vi "Optic Spectrometer.vi"() -> ()   [LabVIEW 2019]
uses:
  <vilib>/DAQmx/write.llb/DAQmx Write (Digital 1D Bool 1Chan 1Samp).vi
  <vilib>/Analysis/baseanly.llb/Mean (DBL).vi
  <vilib>/DAQmx/create/channels.llb/DAQmx Create Channel (DO-Digital Output).vi
  <vilib>/DAQmx/miscellaneous.llb/DAQmx Fill In Error Info.vi
  <vilib>/Analysis/NI_AALBase.lvlib
panel:
  out "End Process":bool
  in  "States":bool[](array[boolean])
  in  "Tab Control":T1(tab)
  out "Gain":dbl=15.0 format="%#_13g"
  in  "Reverse":bool
  in  "Signal Polarity":u16(ring)=1 items=["Module Value", "Real Value"]
  in  "Background Color":u32(colorbox)=16448250
  in  "Plot Color":u32(colorbox)
  in  "Digital Port for Stepper motor":tag="Dev2/port0/line0:3"
  in  "Lamp Spectrum Measuring":bool
  in  "Device name":tag="Dev2"
  in  "Lamp DATA":path=path "C:/Users/Zaza/Google Drive/Projects/Optic Spectrometer/Results/Spectrs Data/Calibrate/250W lamp/IK-5-H1-0.2.txt" caption="Filename"
  in  "Save":bool=TRUE
  in  "Grid":enum32{"Radio Selection 1", "Radio Selection 2"}(radio)=enum."Radio Selection 2"
  in  "File Name":string="Name"
  out "Wavelength[um]":dbl
  out "Baraban":dbl
  in  "Start":dbl=120.0 format="%#_13g"
  in  "Stop":dbl=800.0 format="%#_13g"
  in  "Speed":dbl=100.0
  out "Original Curve":cluster{dbl, dbl}[](graph)=[{0.98, 0.594256}, {0.982, 0.591387}, {0.984, 0.592344}, {0.986, 0.596807}, {0.988, 0.59872}, {0.99, 0.60669}, {0.992, 0.611472}, {0.994, 0.619761}, {0.996, 0.628688}, {0.998, 0.640165}, {1.0, 0.650366}, {1.002, 0.659612}, {1.004, 0.675233}, {1.006, 0.684479}, {1.008, 0.698506}, {1.01, 0.706795}, {1.012, 0.719866}, {1.014, 0.733575}, {1.016, 0.747284}, {1.018, 0.762587}, {1.02, 0.771513}, {1.022, 0.782034}, {1.024, 0.787772}, {1.026, 0.8018}, {1.028, 0.812002}, {1.03, 0.825073}, {1.032, 0.838463}, {1.034, 0.84707}, {1.036, 0.854403}, {1.038, 0.863011}, {1.04, 0.88182}, {1.042, 0.898398}, {1.044, 0.907325}, {1.046, 0.915614}, {1.048, 0.923584}, {1.05, 0.934424}, {1.052, 0.951639}, {1.054, 0.966942}, {1.056, 0.971724}, {1.058, 0.980651}, {1.06, 0.993084}, {1.062, 1.006793}, {1.064, 1.01827}, {1.066, 1.024008}, {1.068, 1.034848}, {1.07, 1.041862}, {1.072, 1.053339}, {1.074, 1.060034}, {1.076, 1.073105}, {1.078, 1.079162}, {1.08, 1.085857}, {1.082, 1.096378}, {1.084, 1.102116}, {1.086, 1.11168}, {1.088, 1.121563}, {1.09, 1.131765}, {1.092, 1.139098}, {1.094, 1.141011}, {1.096, 1.140054}, {1.098, 1.144518}, {1.1, 1.139735}, {1.102, 1.136866}, {1.104, 1.128896}, {1.106, 1.117738}, {1.108, 1.106579}, {1.11, 1.105304}, {1.112, 1.106898}, {1.114, 1.102435}, {1.116, 1.099247}, {1.118, 1.096059}, {1.12, 1.099566}, {1.122, 1.104985}, {1.124, 1.110086}, {1.126, 1.116462}, {1.128, 1.113593}, {1.13, 1.119651}, {1.132, 1.126983}, {1.134, 1.131765}, {1.136, 1.141011}, {1.138, 1.143242}, {1.14, 1.148024}, {1.142, 1.154401}, {1.144, 1.16779}, {1.146, 1.181499}, {1.148, 1.19457}, {1.15, 1.206047}, {1.152, 1.20254}, {1.154, 1.209554}, {1.156, 1.207004}, {1.158, 1.207004}, {1.16, 1.207004}, {1.162, 1.200628}, {1.164, 1.190745}, {1.166, 1.189788}, {1.168, 1.191382}, {1.17, 1.185006}, {1.172, 1.189469}, {1.174, 1.190745}, {1.176, 1.192339}, {1.178, 1.194251}, {1.18, 1.20796}, {1.182, 1.211148}, {1.184, 1.227726}, {1.186, 1.243029}, {1.188, 1.253231}, {1.19, 1.270765}, {1.192, 1.283199}, {1.194, 1.302327}, {1.196, 1.314442}, {1.198, 1.329744}, {1.2, 1.339627}, {1.202, 1.349192}, {1.204, 1.362582}, {1.206, 1.368001}, {1.208, 1.378522}, {1.21, 1.377884}, {1.212, 1.383304}, {1.214, 1.38713}, {1.216, 1.390637}, {1.218, 1.400838}, {1.22, 1.406577}, {1.222, 1.414547}, {1.224, 1.420923}, {1.226, 1.429531}, {1.228, 1.434313}, {1.23, 1.443559}, {1.232, 1.451848}, {1.234, 1.459499}, {1.236, 1.4646}, {1.238, 1.462368}, {1.24, 1.469701}, {1.242, 1.47512}, {1.244, 1.480221}, {1.246, 1.483409}, {1.248, 1.484366}, {1.25, 1.489148}, {1.252, 1.491061}, {1.254, 1.499987}, {1.256, 1.499987}, {1.258, 1.503813}, {1.26, 1.50987}, {1.262, 1.508595}, {1.264, 1.502219}, {1.266, 1.499031}, {1.268, 1.496481}, {1.27, 1.494249}, {1.272, 1.487235}, {1.274, 1.484366}, {1.276, 1.473526}, {1.278, 1.476077}, {1.28, 1.486279}, {1.282, 1.481178}, {1.284, 1.490423}, {1.286, 1.486598}, {1.288, 1.495205}, {1.29, 1.492655}, {1.292, 1.496481}, {1.294, 1.499031}, {1.296, 1.500306}, {1.298, 1.5019}, {1.3, 1.501263}, {1.302, 1.50987}, {1.304, 1.513059}, {1.306, 1.511146}, {1.308, 1.510827}, {1.31, 1.500625}, {1.312, 1.494568}, {1.314, 1.499031}, {1.316, 1.496162}, {1.318, 1.494249}, {1.32, 1.493292}, {1.322, 1.496799}, {1.324, 1.497118}, {1.326, 1.500944}, {1.328, 1.495843}, {1.33, 1.476715}, {1.332, 1.460774}, {1.334, 1.434632}, {1.336, 1.409127}, {1.338, 1.387767}, {1.34, 1.359712}, {1.342, 1.329744}, {1.344, 1.308384}, {1.346, 1.301371}, {1.348, 1.294357}, {1.35, 1.295632}, {1.352, 1.287024}, {1.354, 1.279692}, {1.356, 1.271722}, {1.358, 1.260563}, {1.36, 1.255144}, {1.362, 1.246855}, {1.364, 1.236015}, {1.366, 1.223263}, {1.368, 1.219756}, {1.37, 1.216568}, {1.372, 1.220075}, {1.374, 1.230914}, {1.376, 1.231552}, {1.378, 1.229958}, {1.38, 1.229639}, {1.382, 1.235059}, {1.384, 1.236015}, {1.386, 1.242391}, {1.388, 1.250361}, {1.39, 1.261839}, {1.392, 1.269171}, {1.394, 1.280967}, {1.396, 1.296589}, {1.398, 1.306472}, {1.4, 1.314123}, {1.402, 1.324962}, {1.404, 1.335483}, {1.406, 1.340265}, {1.408, 1.346322}, {1.41, 1.34951}, {1.412, 1.346004}, {1.414, 1.340903}, {1.416, 1.342497}, {1.418, 1.339627}, {1.42, 1.335802}, {1.422, 1.334208}, {1.424, 1.336121}, {1.426, 1.336121}, {1.428, 1.338033}, {1.43, 1.34696}, {1.432, 1.345366}, {1.434, 1.342816}, {1.436, 1.343772}, {1.438, 1.340903}, {1.44, 1.337715}, {1.442, 1.334527}, {1.444, 1.331976}, {1.446, 1.326875}, {1.448, 1.331338}, {1.45, 1.328788}, {1.452, 1.3256}, {1.454, 1.324006}, {1.456, 1.322731}, {1.458, 1.318586}, {1.46, 1.314123}, {1.462, 1.30966}, {1.464, 1.30424}, {1.466, 1.303283}, {1.468, 1.29882}, {1.47, 1.291806}, {1.472, 1.286705}, {1.474, 1.284155}, {1.476, 1.277141}, {1.478, 1.273316}, {1.48, 1.26949}, {1.482, 1.263114}, {1.484, 1.257694}, {1.486, 1.255781}, {1.488, 1.249405}, {1.49, 1.246217}, {1.492, 1.241754}, {1.494, 1.235059}, {1.496, 1.234102}, {1.498, 1.229958}, {1.5, 1.229958}, {1.502, 1.226451}, {1.504, 1.227407}, {1.506, 1.225813}, {1.508, 1.230914}, {1.51, 1.233146}, {1.512, 1.232827}, {1.514, 1.236972}, {1.516, 1.234421}, {1.518, 1.236972}, {1.52, 1.239522}, {1.522, 1.235696}, {1.524, 1.233146}, {1.526, 1.231871}, {1.528, 1.226451}, {1.53, 1.222625}, {1.532, 1.218481}, {1.534, 1.217206}, {1.536, 1.208598}, {1.538, 1.211148}, {1.54, 1.206685}, {1.542, 1.20541}, {1.544, 1.201584}, {1.546, 1.196164}, {1.548, 1.197121}, {1.55, 1.190107}, {1.552, 1.19202}, {1.554, 1.187556}, {1.556, 1.185962}, {1.558, 1.175123}, {1.56, 1.174804}, {1.562, 1.172573}, {1.564, 1.170979}, {1.566, 1.172573}, {1.568, 1.171297}, {1.57, 1.166515}, {1.572, 1.160777}, {1.574, 1.164284}, {1.576, 1.15982}, {1.578, 1.153444}, {1.58, 1.154401}, {1.582, 1.145474}, {1.584, 1.139098}, {1.586, 1.139098}, {1.588, 1.135591}, {1.59, 1.13304}, {1.592, 1.128577}, {1.594, 1.132722}, {1.596, 1.120607}, {1.598, 1.120288}, {1.6, 1.113912}, {1.602, 1.111999}, {1.604, 1.112637}, {1.606, 1.106898}, {1.608, 1.101479}, {1.61, 1.09574}, {1.612, 1.096059}, {1.614, 1.094784}, {1.616, 1.096378}, {1.618, 1.091914}, {1.62, 1.086813}, {1.622, 1.080756}, {1.624, 1.083944}, {1.626, 1.080437}, {1.628, 1.073742}, {1.63, 1.066729}, {1.632, 1.049832}, {1.634, 1.04218}, {1.636, 1.040268}, {1.638, 1.038992}, {1.64, 1.027834}, {1.642, 1.01827}, {1.644, 1.020183}, {1.646, 1.02082}, {1.648, 1.029109}, {1.65, 1.025921}, {1.652, 1.019864}, {1.654, 1.016038}, {1.656, 1.017313}, {1.658, 1.014125}, {1.66, 1.001373}, {1.662, 0.99149}, {1.664, 0.983201}, {1.666, 0.979375}, {1.668, 0.9781}, {1.67, 0.972999}, {1.672, 0.968217}, {1.674, 0.966304}, {1.676, 0.966942}, {1.678, 0.968855}, {1.68, 0.968855}, {1.682, 0.967898}, {1.684, 0.962797}, {1.686, 0.96216}, {1.688, 0.961522}, {1.69, 0.959609}, {1.692, 0.958972}, {1.694, 0.951002}, {1.696, 0.943669}, {1.698, 0.936336}, {1.7, 0.933786}, {1.702, 0.937612}, {1.704, 0.939525}, {1.706, 0.942075}, {1.708, 0.941437}, {1.71, 0.942394}, {1.712, 0.94335}, {1.714, 0.942713}, {1.716, 0.941437}, {1.718, 0.926772}, {1.72, 0.919121}, {1.722, 0.9086}, {1.724, 0.902543}, {1.726, 0.896486}, {1.728, 0.898398}, {1.73, 0.89521}, {1.732, 0.890747}, {1.734, 0.894892}, {1.736, 0.893935}, {1.738, 0.896804}, {1.74, 0.892022}, {1.742, 0.893298}, {1.744, 0.87927}, {1.746, 0.877676}, {1.748, 0.870662}, {1.75, 0.860779}, {1.752, 0.855997}, {1.754, 0.848346}, {1.756, 0.842288}, {1.758, 0.838463}, {1.76, 0.829855}, {1.762, 0.82316}, {1.764, 0.814871}, {1.766, 0.811364}, {1.768, 0.790004}, {1.77, 0.776295}, {1.772, 0.766412}, {1.774, 0.755573}, {1.776, 0.761311}, {1.778, 0.758761}, {1.78, 0.763224}, {1.782, 0.761949}, {1.784, 0.768644}, {1.786, 0.775658}, {1.788, 0.78299}, {1.79, 0.784584}, {1.792, 0.780759}, {1.794, 0.776933}, {1.796, 0.771513}, {1.798, 0.764818}, {1.8, 0.757167}, {1.802, 0.744733}, {1.804, 0.735807}, {1.806, 0.727837}, {1.808, 0.730706}, {1.81, 0.737082}, {1.812, 0.744415}, {1.814, 0.750791}, {1.816, 0.758761}, {1.818, 0.767369}, {1.82, 0.768325}, {1.822, 0.772788}, {1.824, 0.767369}, {1.826, 0.760036}, {1.828, 0.74569}, {1.83, 0.731662}, {1.832, 0.729431}, {1.834, 0.726243}, {1.836, 0.724011}, {1.838, 0.731025}, {1.84, 0.726561}, {1.842, 0.728793}, {1.844, 0.734213}, {1.846, 0.741545}, {1.848, 0.739951}, {1.85, 0.749834}, {1.852, 0.75366}, {1.854, 0.754298}, {1.856, 0.757486}, {1.858, 0.759399}, {1.86, 0.764181}, {1.862, 0.774064}, {1.864, 0.790004}, {1.866, 0.787135}, {1.868, 0.801162}, {1.87, 0.800843}, {1.872, 0.814233}, {1.874, 0.818697}, {1.876, 0.822841}, {1.878, 0.829855}, {1.88, 0.824754}, {1.882, 0.82571}, {1.884, 0.825392}, {1.886, 0.834956}, {1.888, 0.839738}, {1.89, 0.841651}, {1.892, 0.846114}, {1.894, 0.843245}, {1.896, 0.848665}, {1.898, 0.854403}, {1.9, 0.848983}, {1.902, 0.83655}, {1.904, 0.830174}, {1.906, 0.823798}, {1.908, 0.812958}, {1.91, 0.8018}, {1.912, 0.79638}, {1.914, 0.786816}, {1.916, 0.785222}, {1.918, 0.780759}, {1.92, 0.777252}, {1.922, 0.771832}, {1.924, 0.769282}, {1.926, 0.769919}, {1.928, 0.758123}, {1.93, 0.756529}, {1.932, 0.75366}, {1.934, 0.757167}, {1.936, 0.75366}, {1.938, 0.751428}, {1.94, 0.754298}, {1.942, 0.754935}, {1.944, 0.752385}, {1.946, 0.753022}, {1.948, 0.746646}, {1.95, 0.738995}, {1.952, 0.730706}, {1.954, 0.725924}, {1.956, 0.724011}, {1.958, 0.722417}, {1.96, 0.717954}, {1.962, 0.709665}, {1.964, 0.709027}, {1.966, 0.711259}, {1.968, 0.707433}, {1.97, 0.702013}, {1.972, 0.694362}, {1.974, 0.681928}, {1.976, 0.684798}, {1.978, 0.682885}, {1.98, 0.679059}, {1.982, 0.67619}, {1.984, 0.675871}, {1.986, 0.678103}, {1.988, 0.677784}, {1.99, 0.678103}, {1.992, 0.671727}, {1.994, 0.675233}, {1.996, 0.669176}, {1.998, 0.656424}, {2.0, 0.652279}, {2.002, 0.653236}, {2.004, 0.648135}, {2.006, 0.639527}, {2.008, 0.636658}, {2.01, 0.629644}, {2.012, 0.629325}, {2.014, 0.6255}, {2.016, 0.615298}, {2.018, 0.605415}, {2.02, 0.602864}, {2.022, 0.603502}, {2.024, 0.604777}, {2.026, 0.59075}, {2.028, 0.582142}, {2.03, 0.581823}, {2.032, 0.586286}, {2.034, 0.586605}, {2.036, 0.577678}, {2.038, 0.573853}, {2.04, 0.566201}, {2.042, 0.566201}, {2.044, 0.563651}, {2.046, 0.557912}, {2.048, 0.552493}, {2.05, 0.548986}, {2.052, 0.546754}, {2.054, 0.547073}, {2.056, 0.541653}, {2.058, 0.539422}, {2.06, 0.535915}, {2.062, 0.538146}, {2.064, 0.535596}, {2.066, 0.534321}, {2.068, 0.533364}, {2.07, 0.525394}, {2.072, 0.522844}, {2.074, 0.519018}, {2.076, 0.515192}, {2.078, 0.508497}, {2.08, 0.503078}, {2.082, 0.497339}, {2.084, 0.493513}, {2.086, 0.498614}, {2.088, 0.498614}, {2.09, 0.500208}, {2.092, 0.496064}, {2.094, 0.495107}, {2.096, 0.488412}, {2.098, 0.482993}, {2.1, 0.476935}, {2.102, 0.464502}, {2.104, 0.45972}, {2.106, 0.453025}, {2.108, 0.452068}, {2.11, 0.447286}, {2.112, 0.448562}, {2.114, 0.447605}, {2.116, 0.449518}, {2.118, 0.450156}, {2.12, 0.448243}, {2.122, 0.448562}, {2.124, 0.446649}, {2.126, 0.443461}, {2.128, 0.439316}, {2.13, 0.435172}, {2.132, 0.430708}, {2.134, 0.428477}, {2.136, 0.422738}, {2.138, 0.422738}, {2.14, 0.424332}, {2.142, 0.421782}, {2.144, 0.421144}, {2.146, 0.423057}, {2.148, 0.422101}, {2.15, 0.422738}, {2.152, 0.428158}, {2.154, 0.424332}, {2.156, 0.419869}, {2.158, 0.422419}, {2.16, 0.428477}, {2.162, 0.424332}, {2.164, 0.428158}, {2.166, 0.42752}, {2.168, 0.423057}, {2.17, 0.424013}, {2.172, 0.431027}, {2.174, 0.427839}, {2.176, 0.417637}, {2.178, 0.416043}, {2.18, 0.412218}, {2.182, 0.406479}, {2.184, 0.409667}, {2.186, 0.406479}, {2.188, 0.403291}, {2.19, 0.399146}, {2.192, 0.407117}, {2.194, 0.407754}, {2.196, 0.411261}, {2.198, 0.412855}, {2.2, 0.410305}, {2.202, 0.411899}, {2.204, 0.409348}, {2.206, 0.411261}, {2.208, 0.410942}, {2.21, 0.412218}, {2.212, 0.410305}, {2.214, 0.402016}, {2.216, 0.402653}, {2.218, 0.404247}, {2.22, 0.396277}, {2.222, 0.400422}, {2.224, 0.399784}, {2.226, 0.399146}, {2.228, 0.395002}, {2.23, 0.409986}, {2.232, 0.402972}, {2.234, 0.397871}, {2.236, 0.402016}, {2.238, 0.395321}, {2.24, 0.385757}, {2.242, 0.385438}, {2.244, 0.380974}, {2.246, 0.373642}, {2.248, 0.375236}, {2.25, 0.372686}, {2.252, 0.36886}, {2.254, 0.369497}, {2.256, 0.369816}, {2.258, 0.363121}, {2.26, 0.361527}, {2.262, 0.361846}, {2.264, 0.357383}, {2.266, 0.359296}, {2.268, 0.365353}, {2.27, 0.363759}, {2.272, 0.36886}, {2.274, 0.366309}, {2.276, 0.371091}, {2.278, 0.363121}, {2.28, 0.366309}, {2.282, 0.361527}, {2.284, 0.356745}, {2.286, 0.360252}, {2.288, 0.358658}, {2.29, 0.358658}, {2.292, 0.35547}, {2.294, 0.360571}, {2.296, 0.360571}, {2.298, 0.362802}, {2.3, 0.354514}, {2.302, 0.345906}, {2.304, 0.338573}, {2.306, 0.337617}, {2.308, 0.338254}, {2.31, 0.337617}, {2.312, 0.335066}, {2.314, 0.326777}, {2.316, 0.32869}, {2.318, 0.331559}, {2.32, 0.338892}, {2.322, 0.336023}, {2.324, 0.335704}, {2.326, 0.325821}, {2.328, 0.320401}, {2.33, 0.321995}, {2.332, 0.324546}, {2.334, 0.317851}, {2.336, 0.308286}, {2.338, 0.315619}, {2.34, 0.313069}, {2.342, 0.319764}, {2.344, 0.317532}, {2.346, 0.320401}, {2.348, 0.315619}, {2.35, 0.319126}, {2.352, 0.320082}, {2.354, 0.312431}, {2.356, 0.31275}, {2.358, 0.31275}, {2.36, 0.314025}, {2.362, 0.316894}]
  in  "stop":bool
  out "I/I0":cluster{dbl[], dbl[]}(graph)
  out "Normalized":cluster{"Voltage":dbl[], dbl[]}(graph)={"Voltage"=array[691 elements], [1.0, 1.0, 1.0, 1.0, 1.0, 1.0, 1.0, 1.0, 1.0, 1.0, 1.0, 1.0, 1.0, 1.0, 1.0, 1.0, 1.0, 1.0, 1.0, 1.0, 1.0, 1.0, 1.0, 1.0, 1.0, 1.0, 1.0, 1.0, 1.0, 1.0, 1.0, 1.0, 1.0, 1.0, 1.0, 1.0, 1.0, 1.0, 1.0, 1.0, 1.0, 1.0, 1.0, 1.0, 1.0, 1.0, 1.0, 1.0, 1.0, 1.0, 1.0, 1.0, 1.0, 1.0, 1.0, 1.0, 1.0, 1.0, 1.0, 1.0, 1.0, 1.0, 1.0, 1.0, 1.0, 1.0, 1.0, 1.0, 1.0, 1.0, 1.0, 1.0, 1.0, 1.0, 1.0, 1.0, 1.0, 1.0, 1.0, 1.0, 1.0, 1.0, 1.0, 1.0, 1.0, 1.0, 1.0, 1.0, 1.0, 1.0, 1.0, 1.0, 1.0, 1.0, 1.0, 1.0, 1.0, 1.0, 1.0, 1.0, 1.0, 1.0, 1.0, 1.0, 1.0, 1.0, 1.0, 1.0, 1.0, 1.0, 1.0, 1.0, 1.0, 1.0, 1.0, 1.0, 1.0, 1.0, 1.0, 1.0, 1.0, 1.0, 1.0, 1.0, 1.0, 1.0, 1.0, 1.0, 1.0, 1.0, 1.0, 1.0, 1.0, 1.0, 1.0, 1.0, 1.0, 1.0, 1.0, 1.0, 1.0, 1.0, 1.0, 1.0, 1.0, 1.0, 1.0, 1.0, 1.0, 1.0, 1.0, 1.0, 1.0, 1.0, 1.0, 1.0, 1.0, 1.0, 1.0, 1.0, 1.0, 1.0, 1.0, 1.0, 1.0, 1.0, 1.0, 1.0, 1.0, 1.0, 1.0, 1.0, 1.0, 1.0, 1.0, 1.0, 1.0, 1.0, 1.0, 1.0, 1.0, 1.0, 1.0, 1.0, 1.0, 1.0, 1.0, 1.0, 1.0, 1.0, 1.0, 1.0, 1.0, 1.0, 1.0, 1.0, 1.0, 1.0, 1.0, 1.0, 1.0, 1.0, 1.0, 1.0, 1.0, 1.0, 1.0, 1.0, 1.0, 1.0, 1.0, 1.0, 1.0, 1.0, 1.0, 1.0, 1.0, 1.0, 1.0, 1.0, 1.0, 1.0, 1.0, 1.0, 1.0, 1.0, 1.0, 1.0, 1.0, 1.0, 1.0, 1.0, 1.0, 1.0, 1.0, 1.0, 1.0, 1.0, 1.0, 1.0, 1.0, 1.0, 1.0, 1.0, 1.0, 1.0, 1.0, 1.0, 1.0, 1.0, 1.0, 1.0, 1.0, 1.0, 1.0, 1.0, 1.0, 1.0, 1.0, 1.0, 1.0, 1.0, 1.0, 1.0, 1.0, 1.0, 1.0, 1.0, 1.0, 1.0, 1.0, 1.0, 1.0, 1.0, 1.0, 1.0, 1.0, 1.0, 1.0, 1.0, 1.0, 1.0, 1.0, 1.0, 1.0, 1.0, 1.0, 1.0, 1.0, 1.0, 1.0, 1.0, 1.0, 1.0, 1.0, 1.0, 1.0, 1.0, 1.0, 1.0, 1.0, 1.0, 1.0, 1.0, 1.0, 1.0, 1.0, 1.0, 1.0, 1.0, 1.0, 1.0, 1.0, 1.0, 1.0, 1.0, 1.0, 1.0, 1.0, 1.0, 1.0, 1.0, 1.0, 1.0, 1.0, 1.0, 1.0, 1.0, 1.0, 1.0, 1.0, 1.0, 1.0, 1.0, 1.0, 1.0, 1.0, 1.0, 1.0, 1.0, 1.0, 1.0, 1.0, 1.0, 1.0, 1.0, 1.0, 1.0, 1.0, 1.0, 1.0, 1.0, 1.0, 1.0, 1.0, 1.0, 1.0, 1.0, 1.0, 1.0, 1.0, 1.0, 1.0, 1.0, 1.0, 1.0, 1.0, 1.0, 1.0, 1.0, 1.0, 1.0, 1.0, 1.0, 1.0, 1.0, 1.0, 1.0, 1.0, 1.0, 1.0, 1.0, 1.0, 1.0, 1.0, 1.0, 1.0, 1.0, 1.0, 1.0, 1.0, 1.0, 1.0, 1.0, 1.0, 1.0, 1.0, 1.0, 1.0, 1.0, 1.0, 1.0, 1.0, 1.0, 1.0, 1.0, 1.0, 1.0, 1.0, 1.0, 1.0, 1.0, 1.0, 1.0, 1.0, 1.0, 1.0, 1.0, 1.0, 1.0, 1.0, 1.0, 1.0, 1.0, 1.0, 1.0, 1.0, 1.0, 1.0, 1.0, 1.0, 1.0, 1.0, 1.0, 1.0, 1.0, 1.0, 1.0, 1.0, 1.0, 1.0, 1.0, 1.0, 1.0, 1.0, 1.0, 1.0, 1.0, 1.0, 1.0, 1.0, 1.0, 1.0, 1.0, 1.0, 1.0, 1.0, 1.0, 1.0, 1.0, 1.0, 1.0, 1.0, 1.0, 1.0, 1.0, 1.0, 1.0, 1.0, 1.0, 1.0, 1.0, 1.0, 1.0, 1.0, 1.0, 1.0, 1.0, 1.0, 1.0, 1.0, 1.0, 1.0, 1.0, 1.0, 1.0, 1.0, 1.0, 1.0, 1.0, 1.0, 1.0, 1.0, 1.0, 1.0, 1.0, 1.0, 1.0, 1.0, 1.0, 1.0, 1.0, 1.0, 1.0, 1.0, 1.0, 1.0, 1.0, 1.0, 1.0, 1.0, 1.0, 1.0, 1.0, 1.0, 1.0, 1.0, 1.0, 1.0, 1.0, 1.0, 1.0, 1.0, 1.0, 1.0, 1.0, 1.0, 1.0, 1.0, 1.0, 1.0, 1.0, 1.0, 1.0, 1.0, 1.0, 1.0, 1.0, 1.0, 1.0, 1.0, 1.0, 1.0, 1.0, 1.0, 1.0, 1.0, 1.0, 1.0, 1.0, 1.0, 1.0, 1.0, 1.0, 1.0, 1.0, 1.0, 1.0, 1.0, 1.0, 1.0, 1.0, 1.0, 1.0, 1.0, 1.0, 1.0, 1.0, 1.0, 1.0, 1.0, 1.0, 1.0, 1.0, 1.0, 1.0, 1.0, 1.0, 1.0, 1.0, 1.0, 1.0, 1.0, 1.0, 1.0, 1.0, 1.0, 1.0, 1.0, 1.0, 1.0, 1.0, 1.0, 1.0, 1.0, 1.0, 1.0, 1.0, 1.0, 1.0, 1.0, 1.0, 1.0, 1.0, 1.0, 1.0, 1.0, 1.0, 1.0, 1.0, 1.0, 1.0, 1.0, 1.0, 1.0, 1.0, 1.0, 1.0, 1.0, 1.0, 1.0, 1.0, 1.0, 1.0, 1.0, 1.0, 1.0, 1.0, 1.0, 1.0, 1.0, 1.0, 1.0, 1.0, 1.0, 1.0, 1.0, 1.0, 1.0, 1.0, 1.0, 1.0, 1.0, 1.0, 1.0, 1.0, 1.0, 1.0, 1.0, 1.0, 1.0, 1.0, 1.0, 1.0, 1.0, 1.0, 1.0, 1.0, 1.0, 1.0, 1.0, 1.0, 1.0, 1.0, 1.0, 1.0, 1.0, 1.0, 1.0, 1.0, 1.0, 1.0, 1.0, 1.0, 1.0, 1.0, 1.0, 1.0, 1.0, 1.0, 1.0, 1.0, 1.0, 1.0, 1.0, 1.0, 1.0, 1.0, 1.0, 1.0, 1.0]}
  out "Optic spectr Lamp":cluster{"Voltage":dbl[], dbl[]}(graph)
  out "Signal Level":dynamicdata(graph)
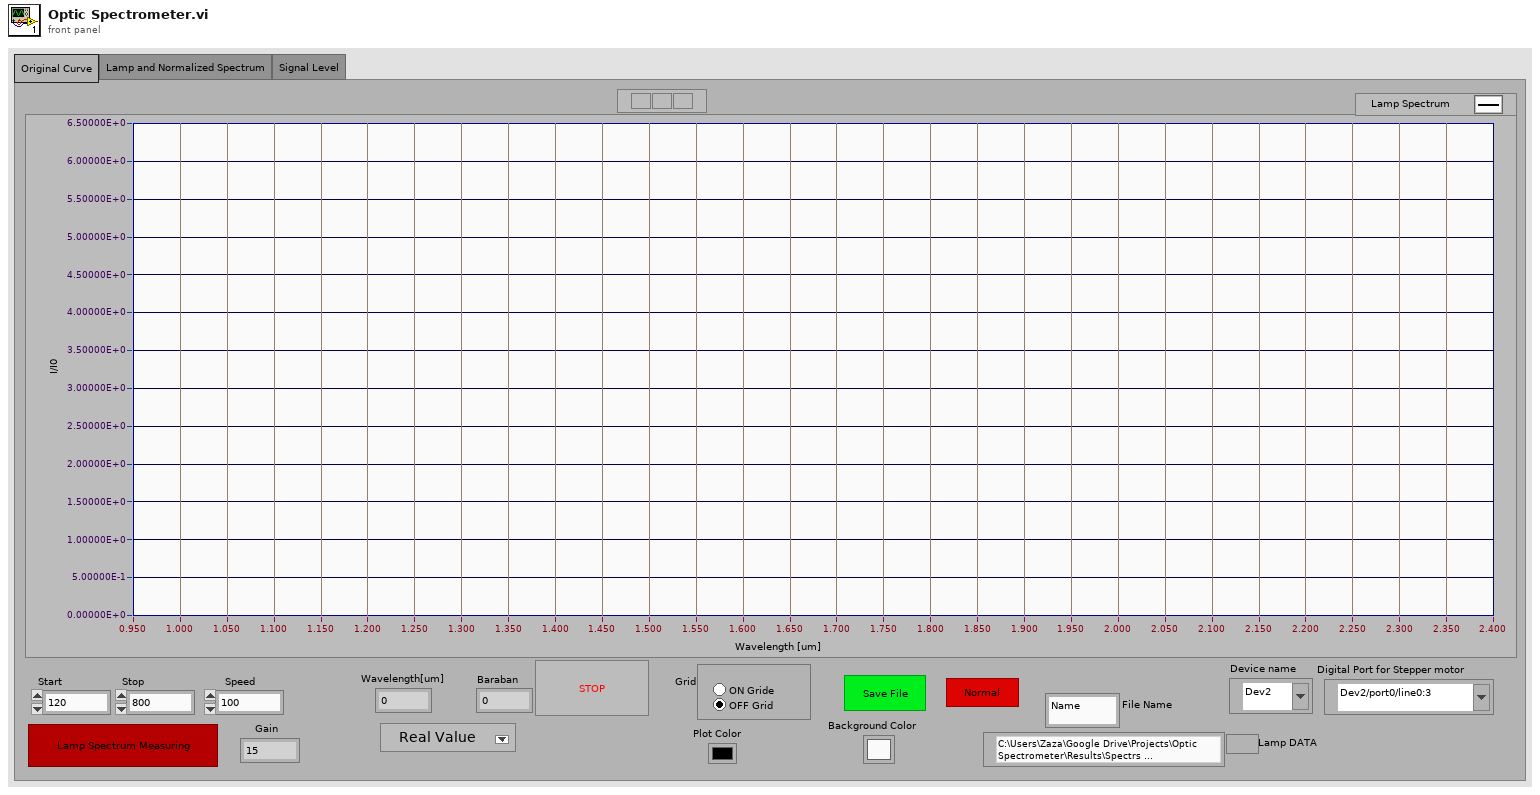
[diagram p1: front panel]
types:
  T1 = enum32{"Original Curve", "Lamp and Normalized Spectrum", "Signal Level"}
  T2 = enum16{"open", "replace", "create", "open or create", "replace or create", "replace or create with confirmation"}
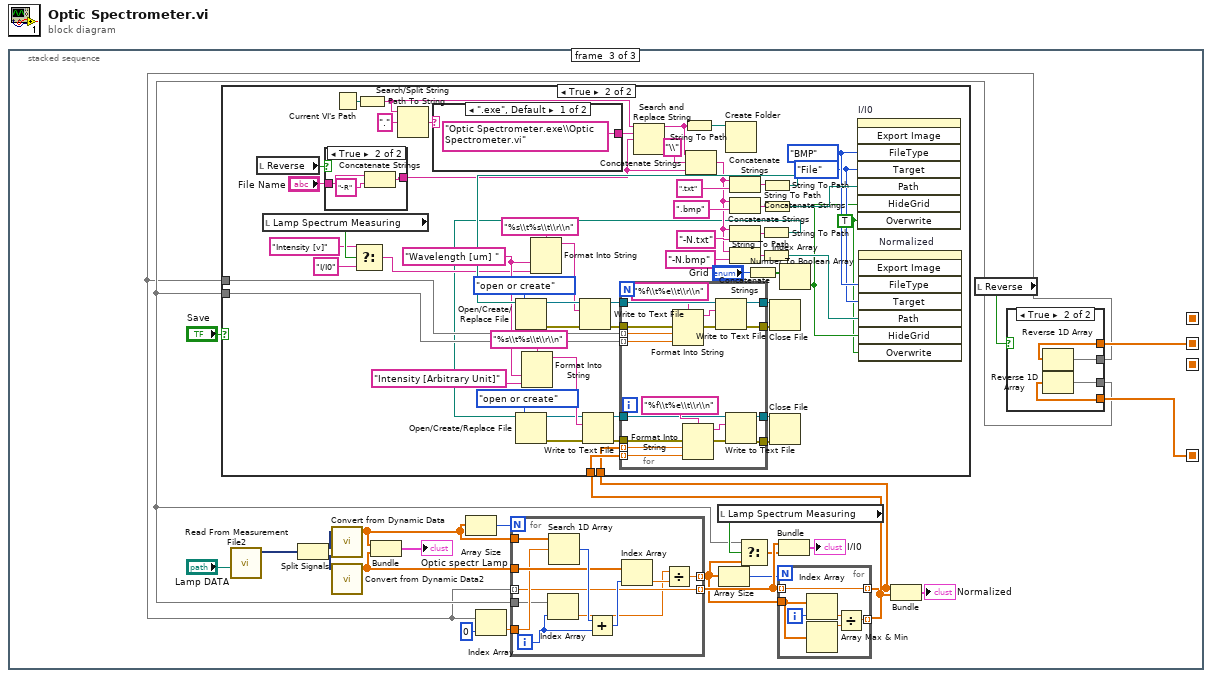
[diagram p0: block diagram]
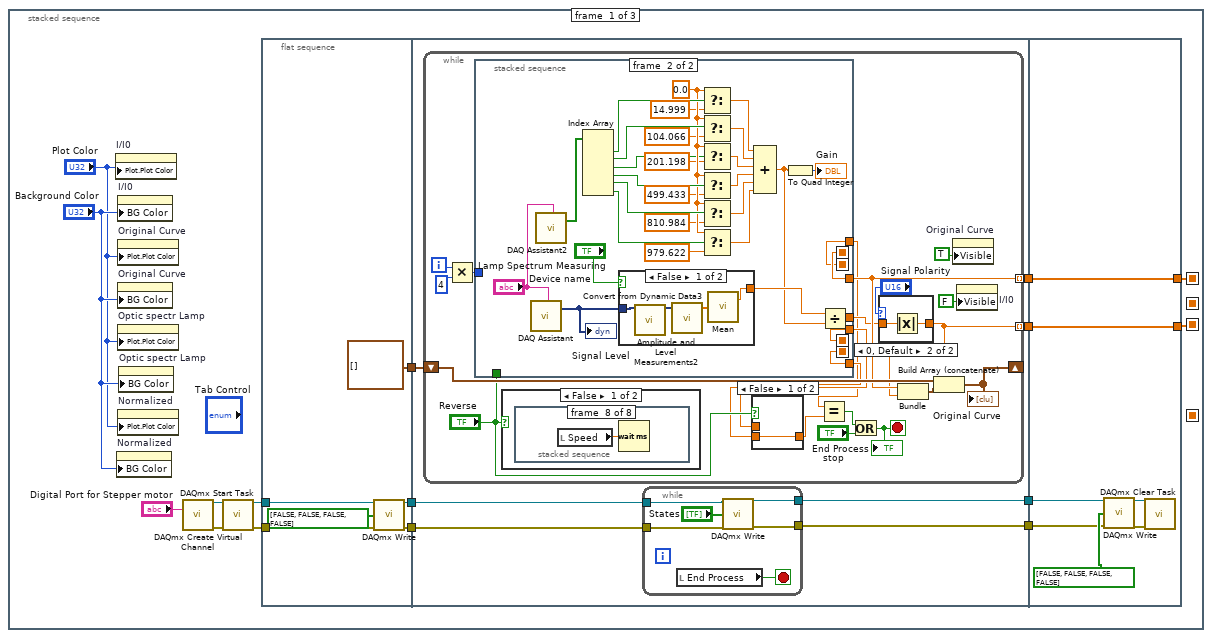
[diagram p2: hidden frame]
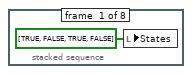
[diagram p4: hidden frame]
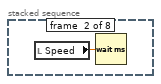
[diagram p5: hidden frame]
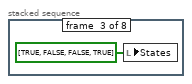
[diagram p6: hidden frame]
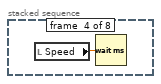
[diagram p7: hidden frame]
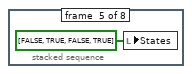
[diagram p8: hidden frame]
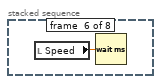
[diagram p9: hidden frame]
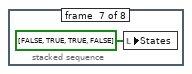
[diagram p10: hidden frame]
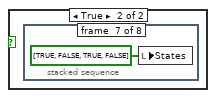
[diagram p11: hidden frame]
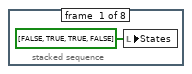
[diagram p12: hidden frame]
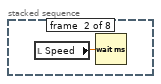
[diagram p13: hidden frame]
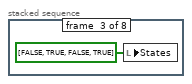
[diagram p14: hidden frame]
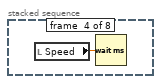
[diagram p15: hidden frame]
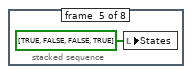
[diagram p16: hidden frame]
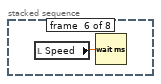
[diagram p17: hidden frame]
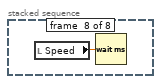
[diagram p18: hidden frame]
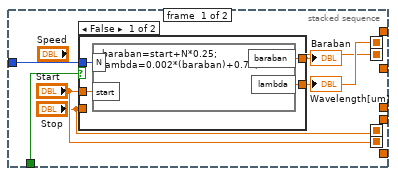
[diagram p20: hidden frame]
diagram:
  n1 = stacked-sequence {
    seq-local: [w16 _ _] -> [_ w145 _]
    seq-local: [w15 _ _] -> [_ w144 _]
    seq-local: [_ w142 _] -> [_ _ w177]
    seq-local: [_ w143 _] -> [_ _ w176]
    frame #0 {
      n2 = property on="I/I0" class="XYGraph (strict)"("Plot.Plot Color"="Plot Color") -> ()  [unwired: 2 in, 2 out]
      n3 = property on="Normalized" class="XYGraph (strict)"("BG Color"="Background Color") -> ()  [unwired: 2 in, 2 out]
      n4 = property on="I/I0" class="XYGraph (strict)"("BG Color"="Background Color") -> ()  [unwired: 2 in, 2 out]
      n5 = property on="Original Curve" class="XYGraph (strict)"("Plot.Plot Color"="Plot Color") -> ()  [unwired: 2 in, 2 out]
      n6 = property on="Original Curve" class="XYGraph (strict)"("BG Color"="Background Color") -> ()  [unwired: 2 in, 2 out]
      n7 = property on="Optic spectr Lamp" class="XYGraph (strict)"("Plot.Plot Color"="Plot Color") -> ()  [unwired: 2 in, 2 out]
      n8 = property on="Normalized" class="XYGraph (strict)"("Plot.Plot Color"="Plot Color") -> ()  [unwired: 2 in, 2 out]
      n9 = property on="Optic spectr Lamp" class="XYGraph (strict)"("BG Color"="Background Color") -> ()  [unwired: 2 in, 2 out]
      n10 = call-poly <vilib>:"DAQmx Create Virtual Channel.vi"("lines"="Digital Port for Stepper motor") -> ("task out"=w3:refnum<k21>, "error out"=w4:errorcluster)  [unwired: 13 in]
      n11 = call <vilib>:"DAQmx Start Task.vi"("task/channels in"=w3, "error in"=w4) -> ("task out"=w2:refnum<k21>, "error out"=w1:errorcluster)  [unwired: 12 in]
      n12 = flat-sequence {
        tunnel: w2 -> [w21]
        tunnel: w1 -> [w20]
        tunnel: [w19] -> w12
        tunnel: [w18] -> w11
        tunnel: [cluster{dbl, "Voltage":dbl}[] []] -> w10
        tunnel: w12 -> [w29]
        tunnel: w11 -> [w28]
        tunnel: [w27] -> w9
        tunnel: [w26] -> w8
        tunnel: w10 -> [w25]
        tunnel: [w24] -> w7
        tunnel: [w23] -> w6
        tunnel: w9 -> [w134]
        tunnel: w8 -> [w133]
        tunnel: [w132] -> w16
        tunnel: w7 -> [w132]
        tunnel: [w131] -> w15
        tunnel: w6 -> [w131]
        frame #0 {
          n13 = call-poly <vilib>:"DAQmx Write.vi"("task/channels in"=w21, "data"=bool[] [FALSE, FALSE, FALSE, FALSE] ("State 1"), "error in"=w20) -> ("task out"=w19:refnum<k21>, "error out"=w18:errorcluster)  [unwired: 10 in, 1 out]
        }
        frame #1 {
          n14 = while {
            shift-right: [w45] -> _
            shift-left: w25 -> [w44]
            tunnel: [w30] -> w23 mode=indexing
            tunnel: [w43] -> w24 mode=indexing
            i -> [w31]
            stop <- w47 stop-if-true
            n15 = Multiply(x=w31, y=4) -> (x*y=w34:i32)
            n16 = stacked-sequence {
              seq-local: [w75 _] -> [_ w115]
              seq-local: ["Start" _] -> [_ w110]
              seq-local: ["Stop" _] -> [_ w111]
              seq-local: [w71 _] -> [_ w109]
              tunnel: w34 -> [w76 _]
              tunnel: [_ w115] -> w43
              tunnel: [_ w112] -> w39
              tunnel: "Reverse" -> [w74 _]
              tunnel: [_ w111] -> w36
              tunnel: [_ w110] -> w35
              tunnel: [_ w109] -> w33
              frame #0 {
                n17 = case shown="False" w74 {
                  tunnel: "Start" -> [w79 w85]
                  tunnel: [w77 w84] -> w71
                  tunnel: w76 -> [w80 w83]
                  tunnel: [w78 w82] -> w75
                  tunnel: "Stop" -> [_ w81]
                  frame False {
                    n18 = formula code="baraban=start+N*0.25;\nlambda=0.002*(baraban)+0.76;"("N"=w80, "start"=w79) -> ("baraban"=w77:dbl, "lambda"=w78:dbl)
                  }
                  frame True {
                    n19 = formula code="baraban=Stop-N*0.25;\nlambda=0.002*(baraban)+0.76;"("N"=w83, "start"=w85, "Stop"=w81) -> ("baraban"=w84:dbl, "lambda"=w82:dbl)
                  }
                }
                "Baraban" <- w71
                "Wavelength[um]" <- w75
              }
              frame #1 {
                w95 = 0.0 ("f")
                n20 = call "DAQ Assistant"("device name"="Device name") -> ("data"=w114:dynamicdata)  [unwired: 16 in, 2 out]
                "Signal Level" <- w114
                n21 = call "DAQ Assistant2"("device name"="Device name") -> ("data"=w101:bool[])  [unwired: 16 in, 2 out]
                n22 = Index Array(array=w101) -> (element #1=w100:bool, element #2=w99:bool, element #3=w88:bool, element #4=w98:bool, element #5=w97:bool, element #6=w96:bool)  [unwired: 6 in]
                n23 = case shown="False" "Lamp Spectrum Measuring" {
                  tunnel: w114 -> [w118 w123]
                  tunnel: [w119 w121] -> w113
                  frame False {
                    n24 = call "Amplitude and Level Measurements2"("Signals"=w118) -> ("Mean (DC)"=w117:dynamicdata)  [unwired: 13 in, 1 out]
                    n25 = call "Convert from Dynamic Data3"("Dynamic Data Type"=w117) -> ("Array"=w120:dbl[])  [unwired: 3 in]
                    n26 = call-poly <vilib>:"Mean.vi"("X"=w120) -> ("mean"=w119:dbl)  [unwired: 1 out]
                  }
                  frame True {
                    n27 = call "Amplitude and Level Measurements"("Signals"=w123) -> ("Peak to Peak"=w124:dynamicdata)  [unwired: 13 in, 1 out]
                    n28 = call "Convert from Dynamic Data4"("Dynamic Data Type"=w124) -> ("Array"=w122:dbl[])  [unwired: 3 in]
                    n29 = call-poly <vilib>:"Mean.vi"("X"=w122) -> ("mean"=w121:dbl)  [unwired: 1 out]
                  }
                }
                n30 = Select(t=w95, s=w100, f=14.999) -> (s? t:f=w107:dbl)
                n31 = Select(t=w95, s=w99, f=104.066) -> (s? t:f=w106:dbl)
                n32 = Select(t=w95, s=w88, f=201.198) -> (s? t:f=w105:dbl)
                n33 = Select(t=w95, s=w98, f=499.433) -> (s? t:f=w104:dbl)
                n34 = Select(t=w95, s=w97, f=810.984) -> (s? t:f=w103:dbl)
                n35 = Select(t=w95, s=w96, f=979.622) -> (s? t:f=w102:dbl)
                n36 = Compound Arithmetic op=ADD(w107, w106, w105, w104, w103, w102) -> (w87:dbl)
                n37 = To Quad Integer(1:w87) -> (0:→"Gain":i64)
                n38 = Divide(x=w113, y=w87) -> (x/y=w112:dbl)
              }
            }
            n39 = case shown="False" "Reverse" {
              frame False {
                n40 = stacked-sequence {
                  frame #0 {
                    n41 = local write "States"(bool[] [TRUE, FALSE, TRUE, FALSE] ("Values")) -> ()
                  }
                  frame #1 {
                    n42 = local read "Speed"() -> (w53:dbl)
                    n43 = Wait (ms)(milliseconds to wait=w53) -> ()  [unwired: 1 out]
                  }
                  frame #2 {
                    n44 = local write "States"(bool[] [TRUE, FALSE, FALSE, TRUE] ("Values")) -> ()
                  }
                  frame #3 {
                    n45 = local read "Speed"() -> (w55:dbl)
                    n46 = Wait (ms)(milliseconds to wait=w55) -> ()  [unwired: 1 out]
                  }
                  frame #4 {
                    n47 = local write "States"(bool[] [FALSE, TRUE, FALSE, TRUE] ("Values")) -> ()
                  }
                  frame #5 {
                    n48 = local read "Speed"() -> (w57:dbl)
                    n49 = Wait (ms)(milliseconds to wait=w57) -> ()  [unwired: 1 out]
                  }
                  frame #6 {
                    n50 = local write "States"(bool[] [FALSE, TRUE, TRUE, FALSE] ("Values")) -> ()
                  }
                  frame #7 {
                    n51 = local read "Speed"() -> (w59:dbl)
                    n52 = Wait (ms)(milliseconds to wait=w59) -> ()  [unwired: 1 out]
                  }
                }
              }
              frame True {
                n53 = stacked-sequence {
                  frame #0 {
                    n54 = local write "States"(bool[] [FALSE, TRUE, TRUE, FALSE] ("Values")) -> ()
                  }
                  frame #1 {
                    n55 = local read "Speed"() -> (w61:dbl)
                    n56 = Wait (ms)(milliseconds to wait=w61) -> ()  [unwired: 1 out]
                  }
                  frame #2 {
                    n57 = local write "States"(bool[] [FALSE, TRUE, FALSE, TRUE] ("Values")) -> ()
                  }
                  frame #3 {
                    n58 = local read "Speed"() -> (w63:dbl)
                    n59 = Wait (ms)(milliseconds to wait=w63) -> ()  [unwired: 1 out]
                  }
                  frame #4 {
                    n60 = local write "States"(bool[] [TRUE, FALSE, FALSE, TRUE] ("Values")) -> ()
                  }
                  frame #5 {
                    n61 = local read "Speed"() -> (w65:dbl)
                    n62 = Wait (ms)(milliseconds to wait=w65) -> ()  [unwired: 1 out]
                  }
                  frame #6 {
                    n63 = local write "States"(bool[] [TRUE, FALSE, TRUE, FALSE] ("Values")) -> ()
                  }
                  frame #7 {
                    n64 = local read "Speed"() -> (w67:dbl)
                    n65 = Wait (ms)(milliseconds to wait=w67) -> ()  [unwired: 1 out]
                  }
                }
              }
            }
            n66 = case shown="False" "Reverse" {
              tunnel: w36 -> [w50 _]
              tunnel: [w50 w51] -> w37
              tunnel: w35 -> [_ w51]
              frame False {
              }
              frame True {
              }
            }
            n67 = Equal?(x=w33, y=w37) -> (x = y?=w49:bool)
            n68 = Or(x=w49, y="stop") -> (x .or. y?=w47:bool)
            "End Process" <- w47
            n69 = case shown="0, Default" "Signal Polarity" {
              tunnel: [w68 w70] -> w30
              tunnel: w39 -> [w68 w69]
              frame 1 {
              }
              frame 0, Default {
                n70 = Absolute Value(x=w69) -> (abs(x)=w70:dbl)
              }
            }
            n71 = Bundle("lambda"=w43, w30) -> (w46:cluster{"lambda":dbl, dbl})  [unwired: 1 in]
            n72 = Build Array (concatenate)(w44, w46) -> (w45:cluster{"lambda":dbl, "Voltage":dbl}[])
            "Original Curve" <- w45
            n73 = property on="Original Curve" class="XYGraph (strict)"("Visible"=TRUE) -> ()  [unwired: 2 in, 2 out]
            n74 = property on="I/I0" class="XYGraph (strict)"("Visible"=FALSE) -> ()  [unwired: 2 in, 2 out]
          }
          n75 = while {
            tunnel: w29 -> [w129]
            tunnel: w28 -> [w126]
            tunnel: [w128] -> w27
            tunnel: [w125] -> w26
            stop <- w130 stop-if-true
            n76 = local read "End Process"() -> (w130:bool)
            n77 = call-poly <vilib>:"DAQmx Write.vi"("task/channels in"=w129, "data"="States", "error in"=w126) -> ("task out"=w128:refnum<k21>, "error out"=w125:errorcluster)  [unwired: 10 in, 1 out]
          }
        }
        frame #2 {
          n78 = call-poly <vilib>:"DAQmx Write.vi"("task/channels in"=w134, "data"=bool[] [FALSE, FALSE, FALSE, FALSE] ("States 2"), "error in"=w133) -> ("task out"=w136:refnum<k21>, "error out"=w135:errorcluster)  [unwired: 10 in, 1 out]
          n79 = call <vilib>:"DAQmx Clear Task.vi"("task in"=w136, "error in"=w135) -> ()  [unwired: 13 in, 1 out]
        }
      }
    }
    frame #1 {
      n80 = local read "Lamp Spectrum Measuring"() -> (w138:bool)
      n81 = for {
        shift-right: [w153] -> _
        shift-left: _ -> [w156]
        shift-right: [w155] -> _
        shift-left: _ -> [w154]
        tunnel: [w152] -> w143 mode=indexing
        tunnel: 8.0 ("Numeric") -> [w153]
        tunnel: w145 -> [w151] mode=indexing
        tunnel: [w151] -> w142 mode=indexing
        tunnel: w144 -> [w150] mode=indexing
        n82 = Array Size(array=w154) -> (size(s)=w157:i32)
        n83 = Not Equal?(x=w153, y=w156) -> (x != y?=w159:bool)
        n84 = Less?(x=w157, y=1) -> (x < y?=w160:bool)
        n85 = Or(x=w159, y=w160) -> (x .or. y?=w161:bool)
        n86 = case shown="False" w161 {
          tunnel: w153 -> [_ w169]
          tunnel: w150 -> [w164 w168]
          tunnel: [w163 w167] -> w155
          tunnel: w154 -> [w166 _]
          frame False {
            n87 = Delete From Array "Delete From Array"(array=w166) -> (array with subset deleted=w165:dbl[])  [unwired: 2 in, 1 out]
            n88 = Insert Into Array "Insert Into Array"(array=w165, index=0, new element=w164) -> (w163:dbl[])
          }
          frame True {
            n89 = Initialize Array "Initialize Array"(w168, w169) -> (w167:dbl[])
          }
        }
        n90 = call-poly <vilib>:"Mean.vi"("X"=w155) -> ("mean"=w152:dbl)  [unwired: 1 out]
      }
      n91 = case shown="False" w138 {
        frame False {
          n92 = property on="I/I0" class="XYGraph (strict)"("YScale.NameLbl.Text"="I/I0" ("Y Scale.Name Label.Text")) -> ()  [unwired: 2 in, 2 out]
          n93 = property on="I/I0" class="XYGraph (strict)"("Plot.Plot Name"="Lamp Spectrum") -> ()  [unwired: 2 in, 2 out]
        }
        frame True {
          n94 = property on="I/I0" class="XYGraph (strict)"("YScale.NameLbl.Text"="Intensity [v]" ("Y Scale.Name Label.Text")) -> ()  [unwired: 2 in, 2 out]
          n95 = property on="I/I0" class="XYGraph (strict)"("Plot.Plot Name"="Intensity") -> ()  [unwired: 2 in, 2 out]
        }
      }
      n96 = property on="I/I0" class="XYGraph (strict)"("Visible"=TRUE) -> ()  [unwired: 2 in, 2 out]
      n97 = property on="Original Curve" class="XYGraph (strict)"("Visible"=FALSE) -> ()  [unwired: 2 in, 2 out]
    }
    frame #2 {
      n98 = call "Read From Measurement File2"("Filename"="Lamp DATA") -> ("Signals"=w180:dynamicdata)  [unwired: 5 in, 5 out]
      n99 = Split Signals(w180) -> (w181:dynamicdata, w182:dynamicdata)  [unwired: 2 in]
      n100 = call "Convert from Dynamic Data"("Dynamic Data Type"=w181) -> ("Array"=w189:dbl[])  [unwired: 3 in]
      n101 = call "Convert from Dynamic Data2"("Dynamic Data Type"=w182) -> ("Array"=w193:dbl[])  [unwired: 3 in]
      n102 = Bundle("Array"=w189, "Array"=w193) -> (→"Optic spectr Lamp":cluster{"Array":dbl[], "Array":dbl[]})  [unwired: 1 in]
      n103 = Array Size(array=w189) -> (size(s)=w194:i32)
      n104 = local read "Lamp Spectrum Measuring"() -> (w183:bool)
      n105 = local read "Reverse"() -> (w175:bool)
      n106 = case shown="True" w175 {
        tunnel: w177 -> [w276 w280]
        tunnel: w176 -> [w275 w279]
        tunnel: [w276 w278] -> w173
        tunnel: [w275 w277] -> w174
        frame False {
        }
        frame True {
          n107 = Reverse 1D Array(array=w280) -> (reversed array=w278:dbl[])
          n108 = Reverse 1D Array(array=w279) -> (reversed array=w277:dbl[])
        }
      }
      n109 = Index Array(array=w173, index=0) -> (element=w192:dbl)
      n110 = for {
        N: w194 -> [_]
        tunnel: w189 -> [w297]
        tunnel: w193 -> [w293]
        tunnel: w192 -> [w292]
        tunnel: [w296] -> w184 mode=indexing
        tunnel: w174 -> [w291]
        tunnel: w173 -> [w290] mode=indexing
        tunnel: [w290] -> w186 mode=indexing
        i -> [w287]
        n111 = Index Array(array=w291, index=w287) -> (element=w288:dbl)
        n112 = Search 1D Array(1D array=w297, element=w292) -> (index of element=w295:i32)  [unwired: 1 in]
        n113 = Add(x=w295, y=w287) -> (x+y=w294:i32)
        n114 = Index Array(array=w293, index=w294) -> (element=w289:dbl)
        n115 = Divide(x=w288, y=w289) -> (x/y=w296:dbl)
      }
      n116 = Array Size(array=w184) -> (size(s)=w178:i32)
      n117 = Select(t=w174, s=w183, f=w184) -> (s? t:f=w185:dbl[])
      n118 = for {
        N: w178 -> [_]
        tunnel: w184 -> [w286]
        tunnel: [w283] -> w171 mode=indexing
        tunnel: w186 -> [w282] mode=indexing
        tunnel: [w282] -> w170 mode=indexing
        i -> [w281]
        n119 = Index Array(array=w286, index=w281) -> (element=w285:dbl)
        n120 = Array Max & Min(array=w286) -> (max value=w284:dbl)  [unwired: 3 out]
        n121 = Divide(x=w285, y=w284) -> (x/y=w283:dbl)
      }
      n122 = case shown="True" "Save" {
        tunnel: w174 -> [_ w200]
        tunnel: w173 -> [_ w199]
        tunnel: w171 -> [_ w198]
        tunnel: w170 -> [_ w197]
        frame False {
        }
        frame True {
          w221 = "Wavelength [um] " ("Signal Name")
          w214 = enum32{"BMP", "EPS", "EMF", "PICT"}."BMP" ("File Type")
          w210 = TRUE ("Always Overwrite")
          w213 = enum32{"File", "Clipboard"}."File" ("Target")
          n123 = local read "Reverse"() -> (w204:bool)
          n124 = local read "Lamp Spectrum Measuring"() -> (w208:bool)
          n125 = case shown="True" w204 {
            tunnel: [w253 w256] -> w202
            tunnel: "File Name" -> [w253 w255]
            frame False {
            }
            frame True {
              n126 = Concatenate Strings(w255, "-R" ("string")) -> (w256:string)
            }
          }
          n127 = Current VI's Path() -> (path=w240:path)
          n128 = Select(t="Intensity [v]" ("Signal Name"), s=w208, f="I/I0" ("Signal Name")) -> (s? t:f=w205:string)
          n129 = Path To String(path=w240) -> (string=w235:string)
          n130 = Search/Split String(string=w235, search string/char (-)=".") -> (match + rest of string=w241:string)  [unwired: 1 in, 2 out]
          n131 = case shown="\".exe\", Default" w241 {
            tunnel: ["Optic Spectrometer.exe\\Optic Spectrometer.vi" ("regular expression") "Optic Spectrometer.vi" ("regular expression")] -> w242
            frame ".exe", Default {
            }
            frame ".vi" {
            }
          }
          n132 = Format Into String(format string="%s\\t%s\\t\\r\\n", w221, "Intensity [Arbitrary Unit]" ("Signal Name")) -> (resulting string=w229:string)  [unwired: 2 in, 1 out]
          n133 = Format Into String(format string="%s\\t%s\\t\\r\\n", w221, w205) -> (resulting string=w243:string)  [unwired: 2 in, 1 out]
          n134 = Search and Replace String(input string=w235, search string=w242, replace string=w202) -> (result string=w238:string)  [unwired: 5 in, 3 out]
          n135 = String To Path(string=w238) -> (path=w239:path)
          n136 = Concatenate Strings(w238, "\\" ("string"), w202) -> (w215:string)
          n137 = Create Folder(path (use dialog)=w239) -> ()  [unwired: 2 in, 3 out]
          n138 = Concatenate Strings(w215, ".txt" ("string")) -> (w233:string)
          n139 = Concatenate Strings(w215, ".bmp" ("string")) -> (w234:string)
          n140 = Concatenate Strings(w215, "-N.txt" ("string")) -> (w216:string)
          n141 = Concatenate Strings(w215, "-N.bmp" ("string")) -> (w217:string)
          n142 = Number To Boolean Array(number="Grid") -> (Boolean array=w252:bool[])
          n143 = String To Path(string=w216) -> (path=w196:path)
          n144 = Open/Create/Replace File(file path (use dialog)=w196, operation (0:open)=T2."open or create") -> (refnum out=w228:refnum<file>, error out=w224:errorcluster)  [unwired: 4 in, 1 out]
          n145 = Write to Text File(file (use dialog)=w228, text=w229, error in=w224) -> (refnum out=w226:refnum<file>, error out=w225:errorcluster)  [unwired: 1 in, 1 out]
          n146 = String To Path(string=w217) -> (path=w212:path)
          n147 = String To Path(string=w233) -> (path=w230:path)
          n148 = Open/Create/Replace File(file path (use dialog)=w230, operation (0:open)=T2."open or create") -> (refnum out=w246:refnum<file>, error out=w245:errorcluster)  [unwired: 4 in, 1 out]
          n149 = Write to Text File(file (use dialog)=w246, text=w243, error in=w245) -> (refnum out=w247:refnum<file>, error out=w248:errorcluster)  [unwired: 1 in, 1 out]
          n150 = for {
            tunnel: w247 -> [w270]
            tunnel: [w272] -> w251
            tunnel: w248 -> [w273]
            tunnel: [w271] -> w250
            tunnel: w226 -> [w266]
            tunnel: w225 -> [w265]
            tunnel: [w264] -> w223
            tunnel: [w263] -> w222
            tunnel: w200 -> [w262] mode=indexing
            tunnel: w199 -> [w261] mode=indexing
            tunnel: w198 -> [w260] mode=indexing
            tunnel: w197 -> [w259] mode=indexing
            n151 = Format Into String(format string="%f\\t%e\\t\\r\\n", w261, w262) -> (resulting string=w274:string)  [unwired: 2 in, 1 out]
            n152 = Format Into String(format string="%f\\t%e\\t\\r\\n", w259, w260) -> (resulting string=w268:string)  [unwired: 2 in, 1 out]
            n153 = Write to Text File(file (use dialog)=w270, text=w274, error in=w273) -> (refnum out=w272:refnum<file>, error out=w271:errorcluster)  [unwired: 1 in, 1 out]
            n154 = Write to Text File(file (use dialog)=w266, text=w268, error in=w265) -> (refnum out=w264:refnum<file>, error out=w263:errorcluster)  [unwired: 1 in, 1 out]
          }
          n155 = String To Path(string=w234) -> (path=w220:path)
          n156 = Close File(refnum=w251, error in=w250) -> ()  [unwired: 2 out]
          n157 = Close File(refnum=w223, error in=w222) -> ()  [unwired: 2 out]
          n158 = Index Array(array=w252) -> (element=w211:bool)  [unwired: 1 in]
          n159 = invoke on="I/I0" class="XYGraph (strict)" method="Export Image"("FileType"=w214, "Target"=w213, "Path"=w220, "HideGrid"=w211, "Overwrite"=w210) -> ()  [unwired: 3 in, 8 out]
          n160 = invoke on="Normalized" class="XYGraph (strict)" method="Export Image"("FileType"=w214, "Target"=w213, "Path"=w212, "HideGrid"=w211, "Overwrite"=w210) -> ()  [unwired: 3 in, 8 out]
        }
      }
      n161 = Bundle(w186, w185) -> (→"I/I0":cluster{dbl[], dbl[]})  [unwired: 1 in]
      n162 = Bundle(w170, w171) -> (→"Normalized":cluster{dbl[], dbl[]})  [unwired: 1 in]
    }
  }
